vi "min_matrix.vi"(10 "Array 3":i32[][](array[numeric]), 11 "Array in":i32[][](array[numeric])) -> (3 "Array out":i32[][](array[numeric]))   [LabVIEW 2020]
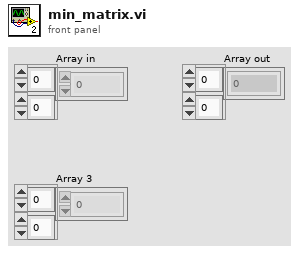
[diagram p1: front panel]
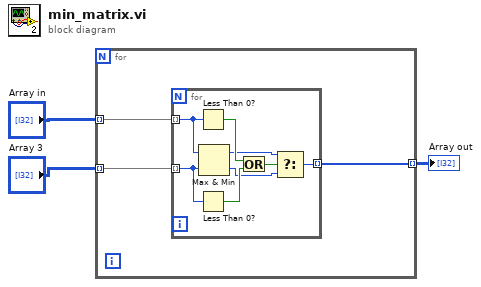
[diagram p0: block diagram]
diagram:
  n1 = for {
    tunnel: "Array 3" -> [w6] mode=indexing
    tunnel: "Array in" -> [w5] mode=indexing
    tunnel: [w4] -> w3 mode=indexing
    n2 = for {
      tunnel: w6 -> [w11] mode=indexing
      tunnel: w5 -> [w12] mode=indexing
      tunnel: [w7] -> w4 mode=indexing
      n3 = Less Than 0?(x=w12) -> (x < 0?=w14:bool)
      n4 = Less Than 0?(x=w11) -> (x < 0?=w13:bool)
      n5 = Max & Min(x=w12, y=w11) -> (max(x,y)=w9:i32, min(x,y)=w8:i32)
      n6 = Or(x=w14, y=w13) -> (x .or. y?=w10:bool)
      n7 = Select(t=w9, s=w10, f=w8) -> (s? t:f=w7:i32)
    }
  }
  "Array out" <- w3
